vi "Set up cameras for acquisition.vi"(8 "error in":errorcluster, 10 "Acquisition cluster":T2={"Save path"=path "D:/DATA_2019", "t frame"=0, "bookmark #"=0, "Z-current"=0, "Channel"=0, "total t frames"=0, "Total bookmarks"=0, "Total z steps"=0, "Total channels"=0, "Gain 1"=100, "Gain 2"=100, "Gain 3"=100, "Gain 4"=100, "Exposure 1"=100.0, "Exposure 2"=100.0, "Exposure 3"=100.0, "Exposure 4"=100.0, "Channel 1"="Red", "Channel 2"="None", "Channel 3"="None", "Channel 4"="None", "Bookmarks?"=FALSE, "Acquisition order"=enum."C-T-Z-B", "t-delay"=0.0, "z-step"=1.0, "Total Images"=1, "Start position"=[], "Piezo radio"=enum."Piezo off", "Piezo Step X"=20.0, "Piezo Step Y"=20.0, "Piezo Step Z"=20.0, "Piezo X current"=0.0, "Piezo Y current"=0.0, "Piezo Z current"=0.0, "LED illumination"=TRUE, "Piezo Amp X"=20.0, "Piezo Amp Y"=20.0, "Piezo Amp Z"=20.0, "Red cropping"={"PosX"=0, "PosY"=0, "Height"=2054, "Width"=2456}, "Green cropping"={"PosX"=0, "PosY"=0, "Height"=2054, "Width"=2456}, "Blue cropping"={"PosX"=0, "PosY"=0, "Height"=2054, "Width"=2456}}, 11 "Instrument cluster":T1) -> (0 "error out":errorcluster)   [LabVIEW 2017]
uses:
  Program flow subVIs/Acquisition cluster.ctl
  Program flow subVIs/Instrument cluster.ctl
  C:/Program Files/National Instruments/LabVIEW 2017/instr.lib/IDS/ueye.NET/uEyeDotNet.dll
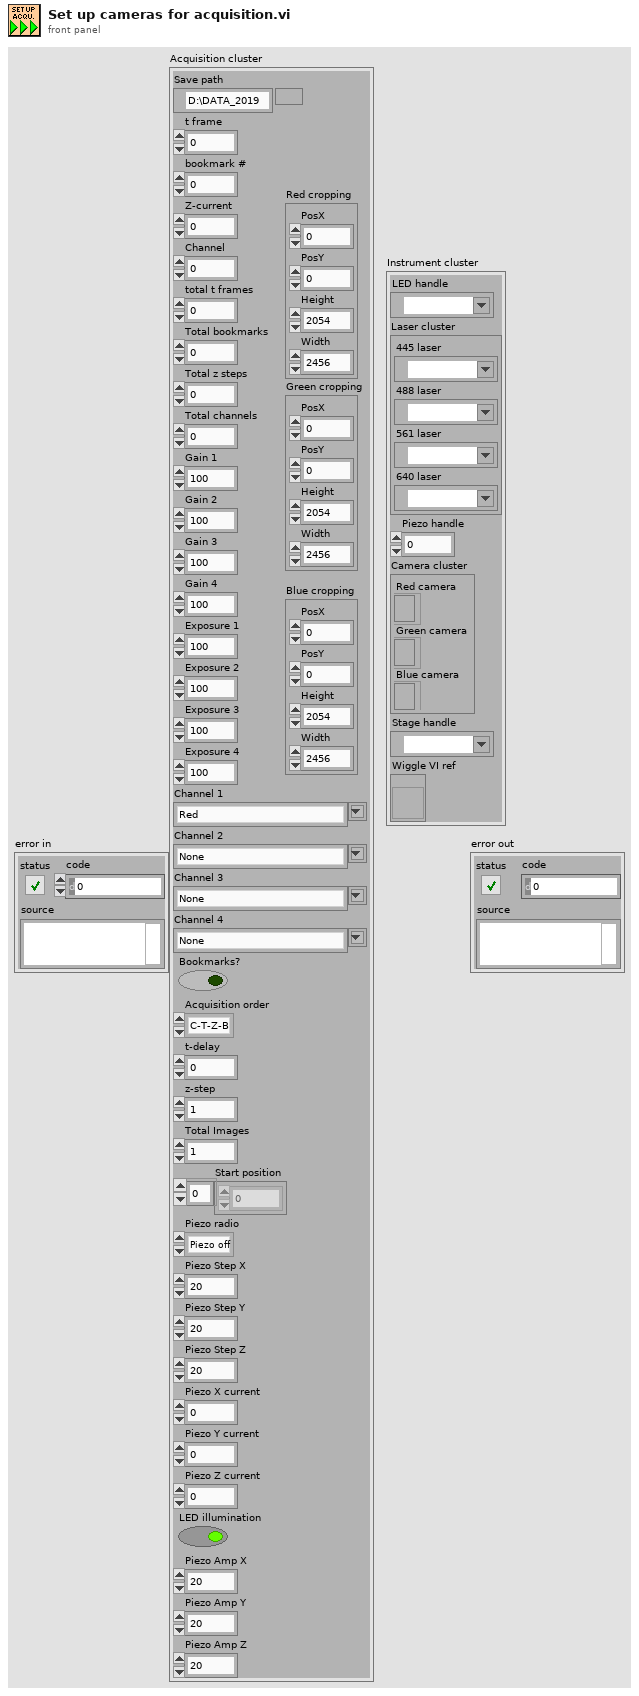
[diagram p1: front panel]
types:
  T1 = typedef "Instrument cluster.ctl" = cluster{"LED handle":refnum<visa-resource-name>, "Laser cluster":cluster{"445 laser":refnum<visa-resource-name>, "488 laser":refnum<visa-resource-name>, "561 laser":refnum<visa-resource-name>, "640 laser":refnum<visa-resource-name>}, "Piezo handle":i32, "Camera cluster":cluster{"Red camera":refnum<k24>, "Green camera":refnum<k24>, "Blue camera":refnum<k24>}, "Stage handle":refnum<visa-resource-name>, "Wiggle VI ref":refnum<vi>}
  T2 = typedef "Acquisition cluster.ctl" = cluster{"Save path":path, "t frame":i32, "bookmark #":i32, "Z-current":i32, "Channel":i32, "total t frames":i32, "Total bookmarks":i32, "Total z steps":i32, "Total channels":i32, "Gain 1":i32, "Gain 2":i32, "Gain 3":i32, "Gain 4":i32, "Exposure 1":dbl, "Exposure 2":dbl, "Exposure 3":dbl, "Exposure 4":dbl, "Channel 1":string, "Channel 2":string, "Channel 3":string, "Channel 4":string, "Bookmarks?":bool, "Acquisition order":enum16{"C-T-Z-B", "C-T-B-Z", "C-Z-T-B", "C-Z-B-T", "C-B-T-Z", "C-B-Z-T", "T-C-Z-B", "T-C-B-Z", "T-Z-C-B", "T-Z-B-C", "T-B-C-Z", "T-B-Z-C", "Z-C-T-B", "Z-C-B-T", "Z-T-C-B", "Z-T-B-C", "Z-B-C-T", "Z-B-T-C", "B-C-T-Z", "B-C-Z-T", "B-Z-C-T", "B-Z-T-C", "B-T-C-Z", "B-T-Z-C"}, "t-delay":dbl, "z-step":dbl, "Total Images":i32, "Start position":dbl[], "Piezo radio":enum32{"Piezo off", "Piezo wiggle", "Piezo step"}, "Piezo Step X":dbl, "Piezo Step Y":dbl, "Piezo Step Z":dbl, "Piezo X current":dbl, "Piezo Y current":dbl, "Piezo Z current":dbl, "LED illumination":bool, "Piezo Amp X":dbl, "Piezo Amp Y":dbl, "Piezo Amp Z":dbl, "Red cropping":cluster{"PosX":i32, "PosY":i32, "Height":i32, "Width":i32}, "Green cropping":cluster{"PosX":i32, "PosY":i32, "Height":i32, "Width":i32}, "Blue cropping":cluster{"PosX":i32, "PosY":i32, "Height":i32, "Width":i32}}
  T3 = cluster{"PosX":i32, "PosY":i32, "Height":i32, "Width":i32}
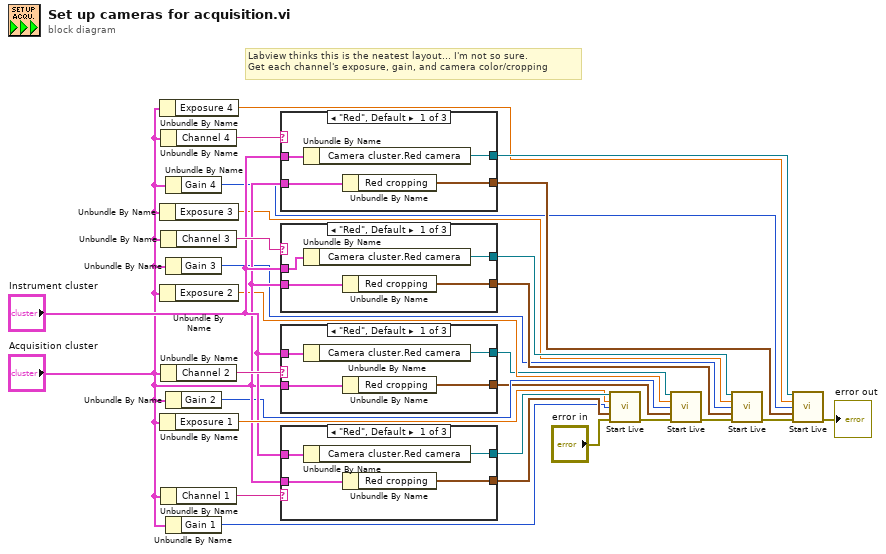
[diagram p0: block diagram]
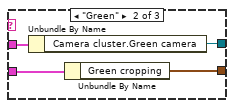
[diagram p2: hidden frame]
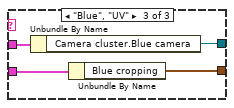
[diagram p3: hidden frame]
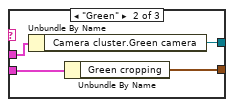
[diagram p4: hidden frame]
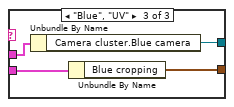
[diagram p5: hidden frame]
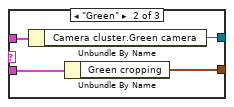
[diagram p6: hidden frame]
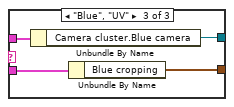
[diagram p7: hidden frame]
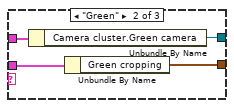
[diagram p8: hidden frame]
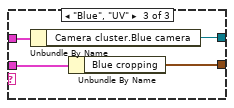
[diagram p9: hidden frame]
diagram:
  # "Labview thinks this is the neatest layout... I'm not so sure.\nGet each channel's exposure, gain, and camera color/cropping"
  n1 = Unbundle By Name("Acquisition cluster") -> ("Exposure 4"=w7:dbl)
  n2 = Unbundle By Name("Acquisition cluster") -> ("Exposure 3"=w1:dbl)
  n3 = Unbundle By Name("Acquisition cluster") -> ("Exposure 2"=w5:dbl)
  n4 = Unbundle By Name("Acquisition cluster") -> ("Exposure 1"=w23:dbl)
  n5 = Unbundle By Name("Acquisition cluster") -> ("Channel 4"=w19:string)
  n6 = Unbundle By Name("Acquisition cluster") -> ("Channel 3"=w20:string)
  n7 = Unbundle By Name("Acquisition cluster") -> ("Channel 2"=w21:string)
  n8 = Unbundle By Name("Acquisition cluster") -> ("Channel 1"=w27:string)
  n9 = Unbundle By Name("Acquisition cluster") -> ("Gain 4"=w8:i32)
  n10 = Unbundle By Name("Acquisition cluster") -> ("Gain 3"=w2:i32)
  n11 = Unbundle By Name("Acquisition cluster") -> ("Gain 2"=w6:i32)
  n12 = Unbundle By Name("Acquisition cluster") -> ("Gain 1"=w24:i32)
  n13 = case shown="\"Red\", Default" w19 {
    tunnel: "Instrument cluster" -> [w31 w35 w39]
    tunnel: "Acquisition cluster" -> [w29 w33 w37]
    tunnel: [w30 w34 w38] -> w16
    tunnel: [w28 w32 w36] -> w15
    frame "Red", Default {
      n14 = Unbundle By Name(w31) -> ("Camera cluster.Red camera"=w30:refnum<k24>)
      n15 = Unbundle By Name(w29) -> ("Red cropping"=w28:T3)
    }
    frame "Green" {
      n16 = Unbundle By Name(w35) -> ("Camera cluster.Green camera"=w34:refnum<k24>)
      n17 = Unbundle By Name(w33) -> ("Green cropping"=w32:T3)
    }
    frame "Blue", "UV" {
      n18 = Unbundle By Name(w39) -> ("Camera cluster.Blue camera"=w38:refnum<k24>)
      n19 = Unbundle By Name(w37) -> ("Blue cropping"=w36:T3)
    }
  }
  n20 = case shown="\"Red\", Default" w20 {
    tunnel: "Instrument cluster" -> [w43 w47 w51]
    tunnel: "Acquisition cluster" -> [w41 w45 w49]
    tunnel: [w42 w46 w50] -> w13
    tunnel: [w40 w44 w48] -> w14
    frame "Red", Default {
      n21 = Unbundle By Name(w43) -> ("Camera cluster.Red camera"=w42:refnum<k24>)
      n22 = Unbundle By Name(w41) -> ("Red cropping"=w40:T3)
    }
    frame "Green" {
      n23 = Unbundle By Name(w47) -> ("Camera cluster.Green camera"=w46:refnum<k24>)
      n24 = Unbundle By Name(w45) -> ("Green cropping"=w44:T3)
    }
    frame "Blue", "UV" {
      n25 = Unbundle By Name(w51) -> ("Camera cluster.Blue camera"=w50:refnum<k24>)
      n26 = Unbundle By Name(w49) -> ("Blue cropping"=w48:T3)
    }
  }
  n27 = case shown="\"Red\", Default" w21 {
    tunnel: "Instrument cluster" -> [w55 w59 w63]
    tunnel: "Acquisition cluster" -> [w53 w57 w61]
    tunnel: [w54 w58 w62] -> w3
    tunnel: [w52 w56 w60] -> w4
    frame "Red", Default {
      n28 = Unbundle By Name(w55) -> ("Camera cluster.Red camera"=w54:refnum<k24>)
      n29 = Unbundle By Name(w53) -> ("Red cropping"=w52:T3)
    }
    frame "Green" {
      n30 = Unbundle By Name(w59) -> ("Camera cluster.Green camera"=w58:refnum<k24>)
      n31 = Unbundle By Name(w57) -> ("Green cropping"=w56:T3)
    }
    frame "Blue", "UV" {
      n32 = Unbundle By Name(w63) -> ("Camera cluster.Blue camera"=w62:refnum<k24>)
      n33 = Unbundle By Name(w61) -> ("Blue cropping"=w60:T3)
    }
  }
  n34 = case shown="\"Red\", Default" w27 {
    tunnel: "Instrument cluster" -> [w67 w71 w75]
    tunnel: "Acquisition cluster" -> [w65 w69 w73]
    tunnel: [w66 w70 w74] -> w26
    tunnel: [w64 w68 w72] -> w25
    frame "Red", Default {
      n35 = Unbundle By Name(w67) -> ("Camera cluster.Red camera"=w66:refnum<k24>)
      n36 = Unbundle By Name(w65) -> ("Red cropping"=w64:T3)
    }
    frame "Green" {
      n37 = Unbundle By Name(w71) -> ("Camera cluster.Green camera"=w70:refnum<k24>)
      n38 = Unbundle By Name(w69) -> ("Green cropping"=w68:T3)
    }
    frame "Blue", "UV" {
      n39 = Unbundle By Name(w75) -> ("Camera cluster.Blue camera"=w74:refnum<k24>)
      n40 = Unbundle By Name(w73) -> ("Blue cropping"=w72:T3)
    }
  }
  n41 = call "Start Live.vi"("Camera reference in"=w26, "Exposure time (ms)"=w23, "Gain in"=w24, "Cropping"=w25, "Error In"="error in") -> ("Error Out"=w12:errorcluster)  [unwired: 9 in, 1 out]
  n42 = call "Start Live.vi"("Camera reference in"=w3, "Exposure time (ms)"=w5, "Gain in"=w6, "Cropping"=w4, "Error In"=w12) -> ("Error Out"=w11:errorcluster)  [unwired: 9 in, 1 out]
  n43 = call "Start Live.vi"("Camera reference in"=w13, "Exposure time (ms)"=w1, "Gain in"=w2, "Cropping"=w14, "Error In"=w11) -> ("Error Out"=w10:errorcluster)  [unwired: 9 in, 1 out]
  n44 = call "Start Live.vi"("Camera reference in"=w16, "Exposure time (ms)"=w7, "Gain in"=w8, "Cropping"=w15, "Error In"=w10) -> ("Error Out"=→"error out":errorcluster)  [unwired: 9 in, 1 out]
